vi "Autonomous Independent.vi"() -> ()   [LabVIEW 2016]
doc: "This VI is called when autonomous begins, and will automatically be terminated when autonomous ends. You can carry out timed or sensor driven robot movement independently without needing to return to the caller."
uses:
  Systems/Global 1.vi
  <vilib>/Rock Robotics/Network Tables/NT Read Number.vi
  Auto_Action.ctl
panel:
  in  "Oscillate effort":dbl=0.25 format="%#_13g"
  out "Auto Mode":dbl=10.0
  in  "Auton_Modes":T2(array[cluster])=[{"Actions"=[{"Effort"=0.55, "Duration"=3.5, "Action"=enum."Nothing", "Encoder"=0.0, "Condition"=FALSE}, {"Effort"=0.0, "Duration"=0.0, "Action"=enum."Nothing", "Encoder"=0.0, "Condition"=FALSE}]}, {"Actions"=[{"Effort"=0.53, "Duration"=1.0, "Action"=enum."Shoot", "Encoder"=6.462, "Condition"=TRUE}, {"Effort"=0.0, "Duration"=3.0, "Action"=enum."Index", "Encoder"=0.0, "Condition"=FALSE}, {"Effort"=0.3, "Duration"=2.0, "Action"=enum."Turn", "Encoder"=38.0, "Condition"=FALSE}, {"Effort"=0.3, "Duration"=5.0, "Action"=enum."Drive", "Encoder"=0.0, "Condition"=TRUE}, {"Effort"=0.25, "Duration"=0.0, "Action"=enum."Nothing", "Encoder"=57.0, "Condition"=FALSE}, {"Effort"=-0.25, "Duration"=0.0, "Action"=enum."Nothing", "Encoder"=0.0, "Condition"=FALSE}, {"Effort"=1.0, "Duration"=0.0, "Action"=enum."Nothing", "Encoder"=0.0, "Condition"=FALSE}, {"Effort"=0.25, "Duration"=0.0, "Action"=enum."Nothing", "Encoder"=0.0, "Condition"=FALSE}]}, {"Actions"=[{"Effort"=0.0, "Duration"=0.1, "Action"=enum."Drive Encoder Reset", "Encoder"=0.0, "Condition"=FALSE}, {"Effort"=0.0, "Duration"=1.0, "Action"=enum."Gyro Reset", "Encoder"=0.0, "Condition"=FALSE}, {"Effort"=0.3, "Duration"=2.5, "Action"=enum."Drive", "Encoder"=1000.0, "Condition"=TRUE}, {"Effort"=1.0, "Duration"=1.0, "Action"=enum."Gear0", "Encoder"=0.0, "Condition"=FALSE}, {"Effort"=1.0, "Duration"=0.0, "Action"=enum."Nothing", "Encoder"=0.0, "Condition"=FALSE}, {"Effort"=1.0, "Duration"=0.5, "Action"=enum."Nothing", "Encoder"=0.0, "Condition"=FALSE}, {"Effort"=0.0, "Duration"=0.0, "Action"=enum."Drive Encoder Reset", "Encoder"=0.0, "Condition"=FALSE}, {"Effort"=0.3, "Duration"=0.5, "Action"=enum."Nothing", "Encoder"=24.0, "Condition"=TRUE}, {"Effort"=0.0, "Duration"=0.0, "Action"=enum."Nothing", "Encoder"=0.0, "Condition"=FALSE}, {"Effort"=-0.2, "Duration"=2.0, "Action"=enum."Drive", "Encoder"=24.0, "Condition"=TRUE}, {"Effort"=0.0, "Duration"=0.0, "Action"=enum."Drive Encoder Reset", "Encoder"=0.0, "Condition"=FALSE}, {"Effort"=-0.25, "Duration"=0.0, "Action"=enum."Nothing", "Encoder"=12.0, "Condition"=FALSE}]}, {"Actions"=[{"Effort"=0.0, "Duration"=0.1, "Action"=enum."Drive Encoder Reset", "Encoder"=6.462, "Condition"=FALSE}, {"Effort"=0.0, "Duration"=0.1, "Action"=enum."Gyro Reset", "Encoder"=0.0, "Condition"=FALSE}, {"Effort"=-0.25, "Duration"=1.0, "Action"=enum."Drive", "Encoder"=6.462, "Condition"=FALSE}, {"Effort"=0.0, "Duration"=0.1, "Action"=enum."Gyro Reset", "Encoder"=0.0, "Condition"=FALSE}, {"Effort"=-0.25, "Duration"=0.0, "Action"=enum."Turn", "Encoder"=0.0, "Condition"=FALSE}, {"Effort"=-0.25, "Duration"=0.0, "Action"=enum."Drive", "Encoder"=7.5, "Condition"=FALSE}, {"Effort"=-1.0, "Duration"=0.0, "Action"=enum."Gear0", "Encoder"=0.0, "Condition"=FALSE}, {"Effort"=0.25, "Duration"=0.0, "Action"=enum."Drive", "Encoder"=3.0, "Condition"=FALSE}]}, {"Actions"=[{"Effort"=0.0, "Duration"=0.1, "Action"=enum."Drive Encoder Reset", "Encoder"=6.462, "Condition"=FALSE}, {"Effort"=0.0, "Duration"=0.1, "Action"=enum."Gyro Reset", "Encoder"=0.0, "Condition"=FALSE}, {"Effort"=-0.25, "Duration"=1.0, "Action"=enum."Drive", "Encoder"=6.462, "Condition"=FALSE}, {"Effort"=0.0, "Duration"=0.1, "Action"=enum."Gyro Reset", "Encoder"=0.0, "Condition"=FALSE}, {"Effort"=-0.25, "Duration"=0.0, "Action"=enum."Turn", "Encoder"=0.0, "Condition"=FALSE}, {"Effort"=-0.25, "Duration"=0.0, "Action"=enum."Drive", "Encoder"=7.5, "Condition"=FALSE}, {"Effort"=-1.0, "Duration"=0.0, "Action"=enum."Gear0", "Encoder"=0.0, "Condition"=FALSE}, {"Effort"=0.25, "Duration"=0.0, "Action"=enum."Drive", "Encoder"=3.0, "Condition"=FALSE}]}, {"Actions"=[{"Effort"=0.0, "Duration"=0.1, "Action"=enum."Drive Encoder Reset", "Encoder"=0.0, "Condition"=FALSE}, {"Effort"=0.0, "Duration"=0.1, "Action"=enum."Gyro Reset", "Encoder"=0.0, "Condition"=FALSE}, {"Effort"=0.25, "Duration"=1.0, "Action"=enum."Drive", "Encoder"=6.462, "Condition"=FALSE}, {"Effort"=1.0, "Duration"=0.1, "Action"=enum."Gyro Reset", "Encoder"=0.0, "Condition"=FALSE}, {"Effort"=0.25, "Duration"=0.0, "Action"=enum."Turn", "Encoder"=0.0, "Condition"=FALSE}, {"Effort"=0.25, "Duration"=0.0, "Action"=enum."Drive", "Encoder"=7.5, "Condition"=FALSE}, {"Effort"=1.0, "Duration"=0.0, "Action"=enum."Gear0", "Encoder"=0.0, "Condition"=FALSE}, {"Effort"=-0.25, "Duration"=0.0, "Action"=enum."Drive", "Encoder"=3.0, "Condition"=FALSE}]}, {"Actions"=[{"Effort"=0.0, "Duration"=0.1, "Action"=enum."Nothing", "Encoder"=0.0, "Condition"=FALSE}, {"Effort"=0.0, "Duration"=0.1, "Action"=enum."Gyro Reset", "Encoder"=0.0, "Condition"=FALSE}, {"Effort"=0.25, "Duration"=5.0, "Action"=enum."Drive", "Encoder"=60000.0, "Condition"=TRUE}, {"Effort"=0.75, "Duration"=1.0, "Action"=enum."Nothing", "Encoder"=0.0, "Condition"=FALSE}, {"Effort"=0.0, "Duration"=1.0, "Action"=enum."Nothing", "Encoder"=0.0, "Condition"=FALSE}, {"Effort"=0.0, "Duration"=0.0, "Action"=enum."Nothing", "Encoder"=0.0, "Condition"=FALSE}]}, {"Actions"=[{"Effort"=0.0, "Duration"=0.5, "Action"=enum."Drive Encoder Reset", "Encoder"=0.0, "Condition"=FALSE}, {"Effort"=0.55, "Duration"=4.25, "Action"=enum."Gyro Reset", "Encoder"=0.0, "Condition"=FALSE}, {"Effort"=-0.5, "Duration"=0.0, "Action"=enum."Drive", "Encoder"=46.0, "Condition"=FALSE}, {"Effort"=0.3, "Duration"=1.0, "Action"=enum."Nothing", "Encoder"=0.0, "Condition"=FALSE}, {"Effort"=0.3, "Duration"=2.0, "Action"=enum."Vision Correction", "Encoder"=76.6, "Condition"=FALSE}, {"Effort"=-0.25, "Duration"=1.0, "Action"=enum."Drive", "Encoder"=18.5, "Condition"=TRUE}, {"Effort"=1.0, "Duration"=0.0, "Action"=enum."Gear0", "Encoder"=0.0, "Condition"=FALSE}, {"Effort"=0.3, "Duration"=1.3, "Action"=enum."Drive", "Encoder"=30.0, "Condition"=TRUE}, {"Effort"=0.0, "Duration"=0.0, "Action"=enum."Nothing", "Encoder"=0.0, "Condition"=FALSE}, {"Effort"=0.03, "Duration"=0.0, "Action"=enum."Turn", "Encoder"=0.0, "Condition"=FALSE}, {"Effort"=0.0, "Duration"=0.0, "Action"=enum."Drive", "Encoder"=0.0, "Condition"=FALSE}]}, {"Actions"=[{"Effort"=0.0, "Duration"=0.0, "Action"=enum."Nothing", "Encoder"=0.0, "Condition"=FALSE}]}, {"Actions"=[{"Effort"=0.0, "Duration"=2.5, "Action"=enum."Shoot", "Encoder"=0.0, "Condition"=FALSE}, {"Effort"=0.0, "Duration"=5.0, "Action"=enum."Index", "Encoder"=0.0, "Condition"=FALSE}, {"Effort"=0.25, "Duration"=3.5, "Action"=enum."Nothing", "Encoder"=88.0, "Condition"=FALSE}, {"Effort"=1.0, "Duration"=1.0, "Action"=enum."Nothing", "Encoder"=0.0, "Condition"=FALSE}, {"Effort"=1.0, "Duration"=1.0, "Action"=enum."Nothing", "Encoder"=0.0, "Condition"=FALSE}, {"Effort"=1.0, "Duration"=0.5, "Action"=enum."Nothing", "Encoder"=0.0, "Condition"=FALSE}, {"Effort"=0.0, "Duration"=0.0, "Action"=enum."Nothing", "Encoder"=0.0, "Condition"=FALSE}, {"Effort"=-0.25, "Duration"=0.0, "Action"=enum."Nothing", "Encoder"=3.0, "Condition"=FALSE}, {"Effort"=0.0, "Duration"=0.0, "Action"=enum."Nothing", "Encoder"=0.0, "Condition"=FALSE}, {"Effort"=0.25, "Duration"=0.0, "Action"=enum."Nothing", "Encoder"=24.0, "Condition"=FALSE}, {"Effort"=0.0, "Duration"=0.0, "Action"=enum."Nothing", "Encoder"=0.0, "Condition"=FALSE}, {"Effort"=-0.25, "Duration"=0.0, "Action"=enum."Nothing", "Encoder"=12.0, "Condition"=FALSE}]}, {"Actions"=[{"Effort"=0.0, "Duration"=0.1, "Action"=enum."Drive Encoder Reset", "Encoder"=0.0, "Condition"=FALSE}, {"Effort"=0.0, "Duration"=1.0, "Action"=enum."Gyro Reset", "Encoder"=0.0, "Condition"=FALSE}, {"Effort"=0.3, "Duration"=1.4, "Action"=enum."Drive", "Encoder"=88.0, "Condition"=TRUE}, {"Effort"=0.3, "Duration"=4.0, "Action"=enum."Turn", "Encoder"=2.0, "Condition"=FALSE}, {"Effort"=1.0, "Duration"=1.0, "Action"=enum."Nothing", "Encoder"=0.0, "Condition"=FALSE}, {"Effort"=1.0, "Duration"=0.5, "Action"=enum."Nothing", "Encoder"=0.0, "Condition"=FALSE}, {"Effort"=0.0, "Duration"=0.0, "Action"=enum."Nothing", "Encoder"=0.0, "Condition"=FALSE}, {"Effort"=-0.25, "Duration"=0.0, "Action"=enum."Nothing", "Encoder"=3.0, "Condition"=FALSE}, {"Effort"=0.0, "Duration"=0.0, "Action"=enum."Nothing", "Encoder"=0.0, "Condition"=FALSE}, {"Effort"=0.25, "Duration"=0.0, "Action"=enum."Nothing", "Encoder"=24.0, "Condition"=FALSE}, {"Effort"=0.0, "Duration"=0.0, "Action"=enum."Nothing", "Encoder"=0.0, "Condition"=FALSE}, {"Effort"=-0.25, "Duration"=0.0, "Action"=enum."Nothing", "Encoder"=12.0, "Condition"=FALSE}]}, {"Actions"=[{"Effort"=0.0, "Duration"=1.0, "Action"=enum."Drive Encoder Reset", "Encoder"=0.0, "Condition"=FALSE}, {"Effort"=0.0, "Duration"=1.0, "Action"=enum."Shoot", "Encoder"=0.0, "Condition"=FALSE}, {"Effort"=0.25, "Duration"=5.0, "Action"=enum."Index", "Encoder"=88.0, "Condition"=FALSE}, {"Effort"=1.0, "Duration"=1.0, "Action"=enum."Nothing", "Encoder"=0.0, "Condition"=FALSE}, {"Effort"=1.0, "Duration"=1.0, "Action"=enum."Nothing", "Encoder"=0.0, "Condition"=FALSE}, {"Effort"=1.0, "Duration"=0.5, "Action"=enum."Nothing", "Encoder"=0.0, "Condition"=FALSE}, {"Effort"=0.0, "Duration"=0.0, "Action"=enum."Nothing", "Encoder"=0.0, "Condition"=FALSE}, {"Effort"=-0.25, "Duration"=0.0, "Action"=enum."Nothing", "Encoder"=3.0, "Condition"=FALSE}, {"Effort"=0.0, "Duration"=0.0, "Action"=enum."Nothing", "Encoder"=0.0, "Condition"=FALSE}, {"Effort"=0.25, "Duration"=0.0, "Action"=enum."Nothing", "Encoder"=24.0, "Condition"=FALSE}, {"Effort"=0.0, "Duration"=0.0, "Action"=enum."Nothing", "Encoder"=0.0, "Condition"=FALSE}, {"Effort"=-0.25, "Duration"=0.0, "Action"=enum."Nothing", "Encoder"=12.0, "Condition"=FALSE}]}, {"Actions"=[{"Effort"=0.0, "Duration"=0.1, "Action"=enum."Drive Encoder Reset", "Encoder"=0.0, "Condition"=FALSE}, {"Effort"=0.0, "Duration"=1.0, "Action"=enum."Gyro Reset", "Encoder"=0.0, "Condition"=FALSE}, {"Effort"=0.3, "Duration"=1.4, "Action"=enum."Drive", "Encoder"=88.0, "Condition"=TRUE}, {"Effort"=0.3, "Duration"=4.0, "Action"=enum."Turn", "Encoder"=0.0, "Condition"=FALSE}, {"Effort"=1.0, "Duration"=1.0, "Action"=enum."Nothing", "Encoder"=0.0, "Condition"=FALSE}, {"Effort"=1.0, "Duration"=0.5, "Action"=enum."Nothing", "Encoder"=0.0, "Condition"=FALSE}, {"Effort"=0.0, "Duration"=0.0, "Action"=enum."Nothing", "Encoder"=0.0, "Condition"=FALSE}, {"Effort"=0.3, "Duration"=0.5, "Action"=enum."Nothing", "Encoder"=24.0, "Condition"=TRUE}, {"Effort"=0.0, "Duration"=0.0, "Action"=enum."Nothing", "Encoder"=0.0, "Condition"=FALSE}, {"Effort"=-0.2, "Duration"=2.0, "Action"=enum."Nothing", "Encoder"=24.0, "Condition"=TRUE}, {"Effort"=0.0, "Duration"=0.0, "Action"=enum."Nothing", "Encoder"=0.0, "Condition"=FALSE}, {"Effort"=-0.25, "Duration"=0.0, "Action"=enum."Nothing", "Encoder"=12.0, "Condition"=FALSE}]}]
  # "Nothing"
  # "Boiler Right Right side gear"
  # "Middle Gear"
  # "Boiler Right Left Side Gear"
  # "Boiler Left RightSide Gear"
  # "Boiler Left Left Side Gear"
  # "Drive"
  # "Vision Correction"
  # "Hopper"
  # "10 ball"
  # "Farside"
  # "Boilerside-10 ball"
  # "Auto 5"
  # "Auto 6"
  # "Auto 6"
  # "Auto 7"
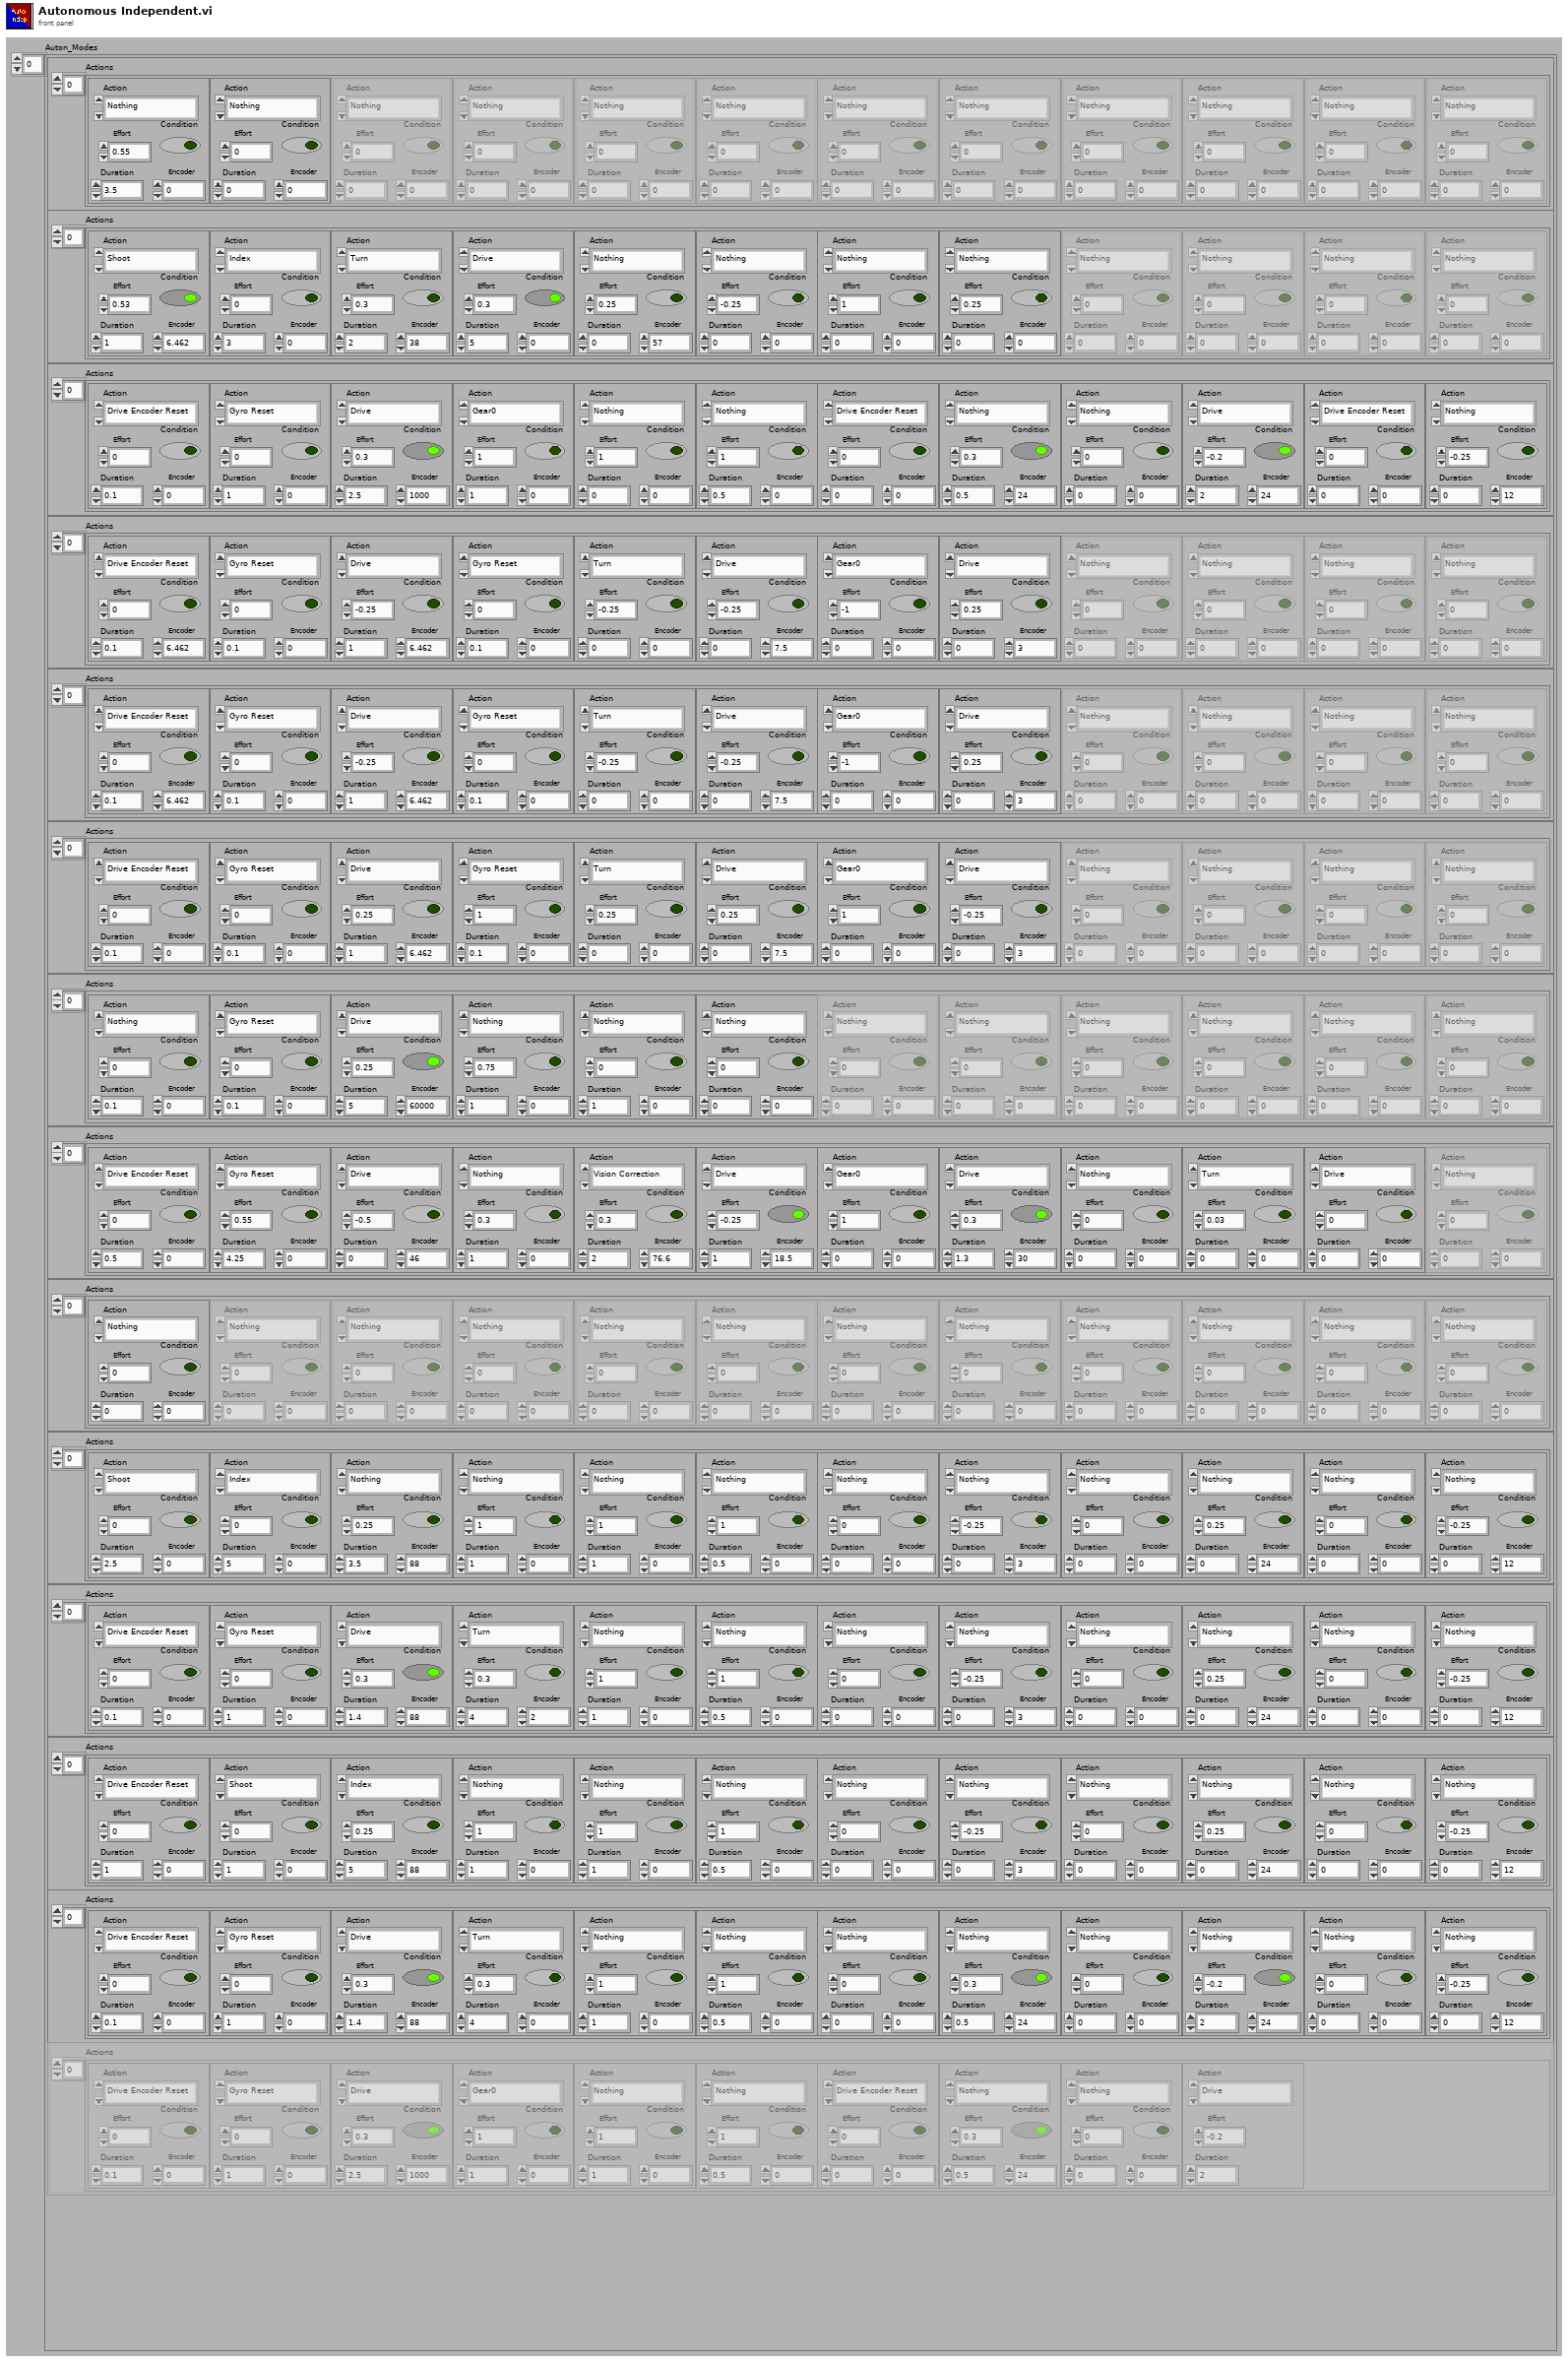
[diagram p1: front panel]
types:
  T1 = typedef "Auto_Action.ctl" = enum16{"Nothing", "Drive", "Vision Correction", "Turn", "Gear0", "Gear1", "Climb", "Intake", "Index", "Shoot", "Test", "Drive Encoder Reset", "Gyro Reset"}
  T2 = cluster{"Actions":cluster{"Effort":dbl, "Duration":dbl, "Action":T1, "Encoder":dbl, "Condition":bool}[]}[]
  T3 = cluster{"Actions":cluster{"Effort":dbl, "Duration":dbl, "Action":T1, "Encoder":dbl, "Condition":bool}[]}
  T4 = cluster{"Effort":dbl, "Duration":dbl, "Action":T1, "Encoder":dbl, "Condition":bool}[]
  T5 = typedef "WPI_MotorControlDeviceRef.ctl" = cluster{"DeviceStatus":errorcluster, "Type":T6, "PWM":cluster{"PWM Channel":T7, "DeadBand":T8}, "CAN":cluster{"Device Number":u8, "SetOutput VI Ref":variant, "GetOutput VI Ref":variant, "Enable VI Ref":variant, "Disable VI Ref":variant, "Data":variant}, "Invert":bool}
  T6 = typedef "WPI_MotorControlType.ctl" = enum16{"PWM", "CAN"}
  T7 = typedef "FPGA_DIOPWMChannel.ctl" = enum8{"PWM 0", "PWM 1", "PWM 2", "PWM 3", "PWM 4", "PWM 5", "PWM 6", "PWM 7", "PWM 8", "PWM 9", "PWM MXP 0", "PWM MXP 1", "PWM MXP 2", "PWM MXP 3", "PWM MXP 4", "PWM MXP 5", "PWM MXP 6", "PWM MXP 7", "PWM MXP 8", "PWM MXP 9", "Invalid"}
  T8 = typedef "WPI_PWMDeadband.ctl" = cluster{"Name":string, "maxPositivePwm":i32, "minPositivePwm":i32, "centerPwm":i32, "maxNegativePwm":i32, "minNegativePwm":i32, "angularRange":u16}
  T9 = typedef "WPI_CANTalonSRX_GlobalStatus.ctl" = cluster{"Applied Throttle":dbl, "Module Enabled":bool, "CAN Error":errorcluster, "Closed Loop Error":dbl, "Forward Limit Switch Closed":bool, "Reverse Limit Switch Closed":bool, "Sensor Position":dbl, "Sensor Velocity":dbl, "Current":dbl, "Sticky Fault - Over Temp":bool, "Sticky Fault - Under Voltage":bool, "Sticky Fault - Forward Limit":bool, "Sticky Fault - Reverse Limit":bool, "Sticky Fault - Forward Soft Limit":bool, "Sticky Fault - Reverse Soft Limit":bool, "Brake is Enabled":bool, "Encoder Position":dbl, "Encoder Velocity":dbl, "Encoder Index Count":dbl, "Encoder A Pin State":bool, "Encoder B Pin State":bool, "Encoder Index Pin State":bool, "Analog In":dbl, "Analog In Velocity":dbl, "Temperature (C)":dbl, "Battery Voltage":dbl, "Control 5 Is Supported":bool, "Current Profile Slot Select":dbl, "Pos Div 8":bool, "Vel Div 4":bool, "Pulse Width Position":i32, "Pulse Width Velocity":i32, "Pulse Width Rise To Rise (us)":i32, "Pulse Width Rise To Fall (us)":i32, "Mot Prof Active Is Under Run":bool, "Mot Prof Active Has Under Run":bool, "Mot Prof Active Is Last":bool, "Mot Prof Active Velocity Only":bool, "Mot Prof Active Is Valid":bool, "Mot Prof Buffer Is Full":bool, "Mot Prof Active Profile Slot Select":i32, "Mot Prof NextID":i32, "Mot Prof Count":i32, "Mot Prof Active Velocity":dbl, "Mot Prof Active Position":dbl, "Mot Prof Output Enable":i32}
  T10 = typedef "WPI_GyroDevRef.ctl" = cluster{"DevStatus":errorcluster, "Analog Channel":T11, "Offset":dbl, "Gain (VoltsPerDegree/Second)":dbl, "Gyro Type":enum16{"Analog", "XRS450"}, "Handle":i32, "SPI Bus":T12, "Device Found":bool, "Sample Rate":dbl, "Calibrate On Open":bool}
  T11 = typedef "FPGA_AIChannel.ctl" = enum8{"AI 0", "AI 1", "AI 2", "AI 3", "AI MXP 0", "AI MXP 1", "AI MXP 2", "AI MXP 3", "Invalid"}
  T12 = typedef "spi_bus.ctl" = enum16{"SPI On-Board, CS0", "SPI On-Board, CS1", "SPI On-Board, CS2", "SPI On-Board, CS3", "SPI MXP", "Invalid"}
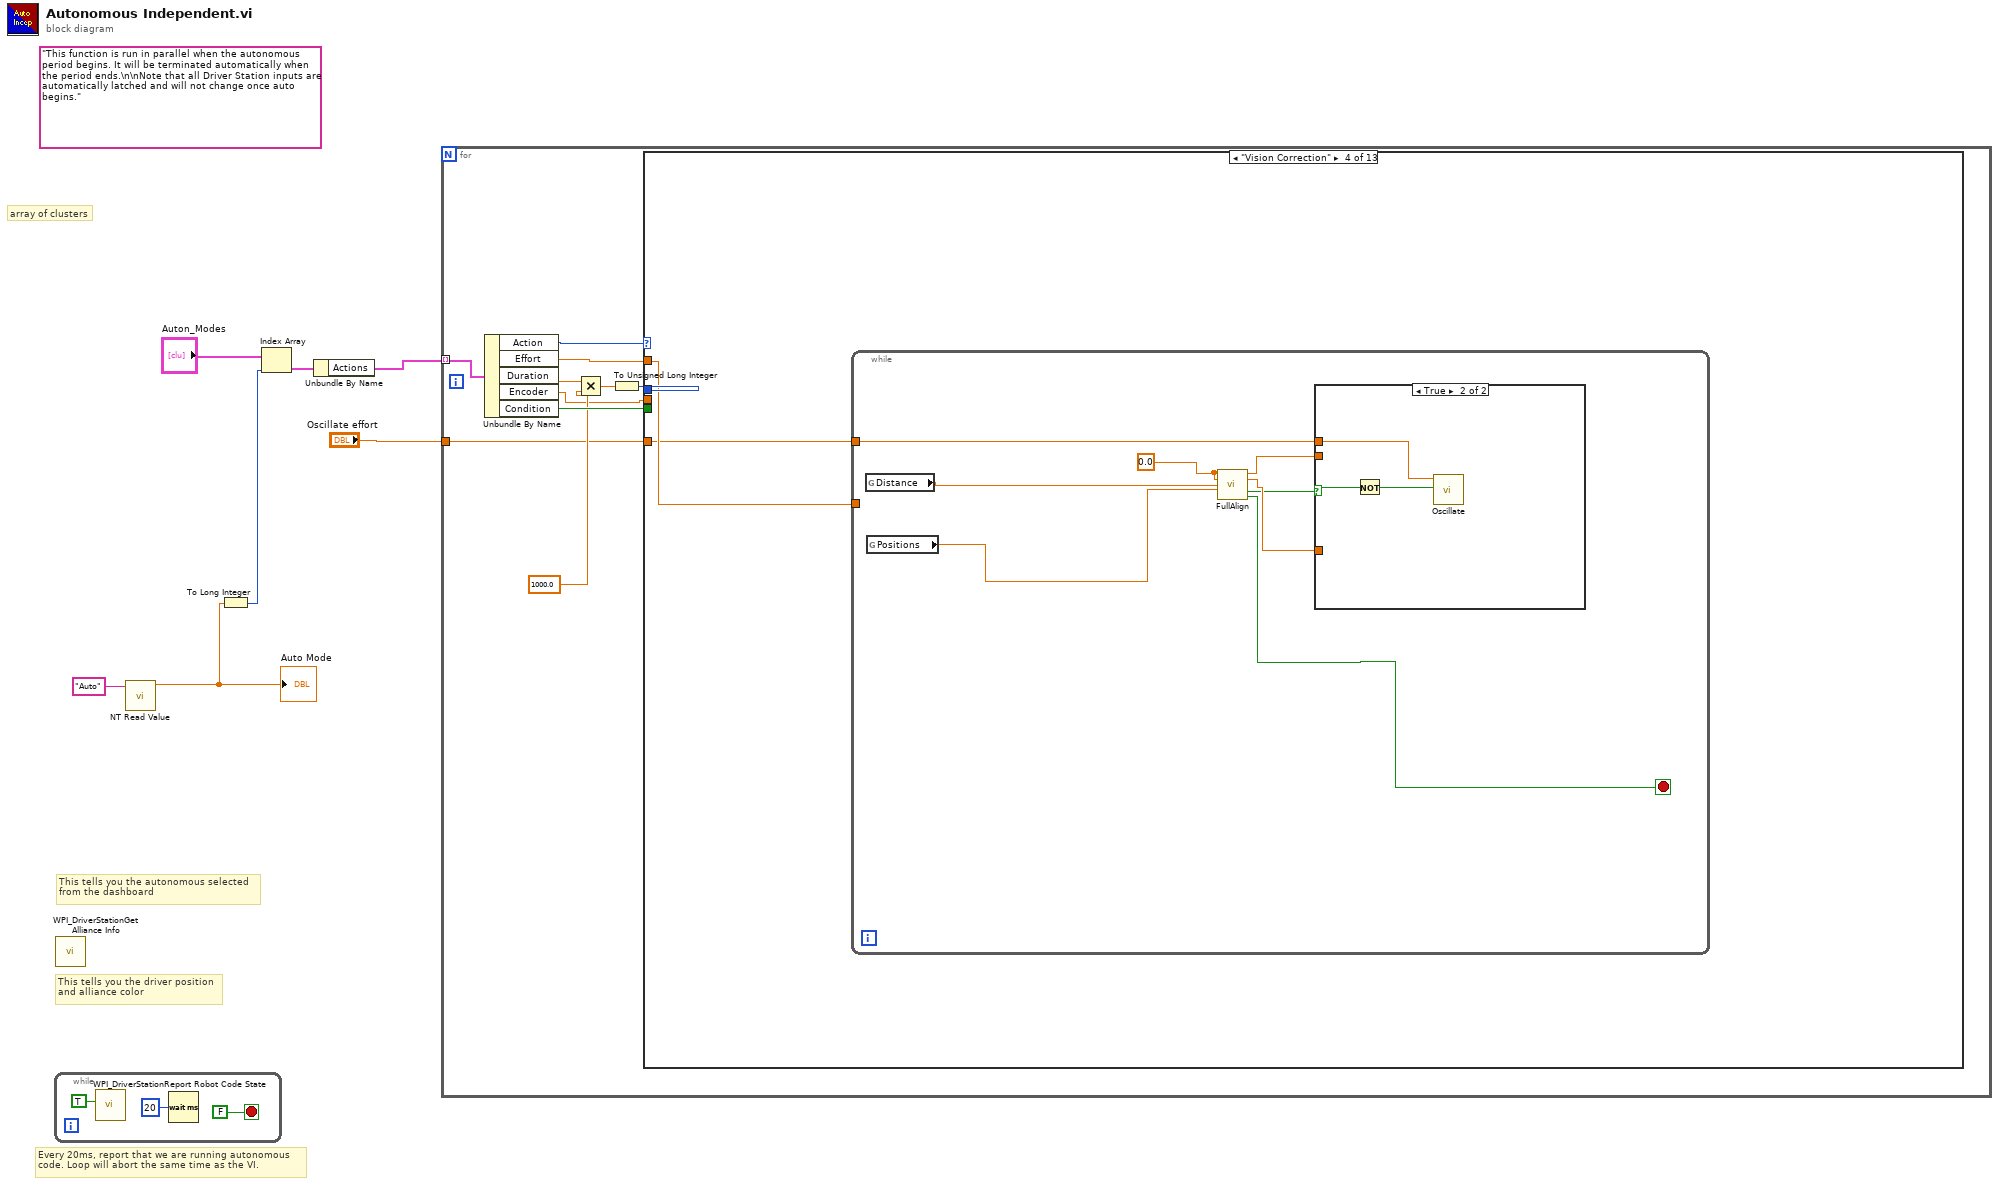
[diagram p0: block diagram]
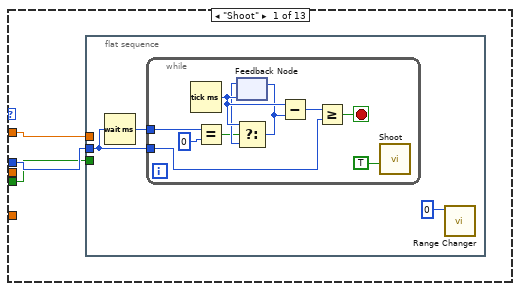
[diagram p2: hidden frame]
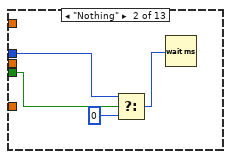
[diagram p3: hidden frame]
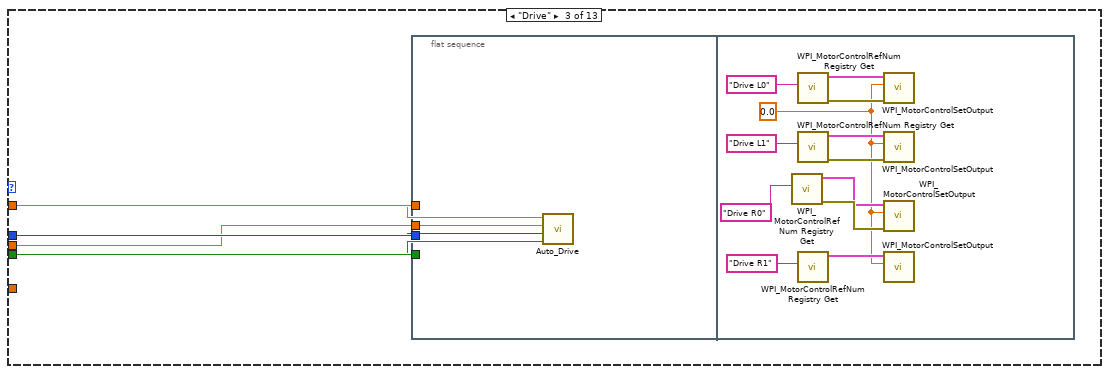
[diagram p4: hidden frame]
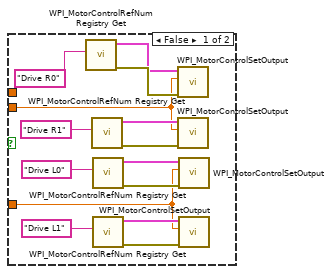
[diagram p5: hidden frame]
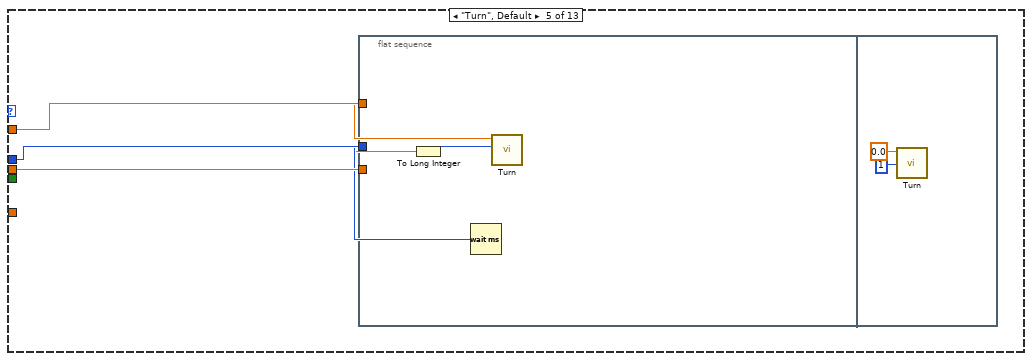
[diagram p6: hidden frame]
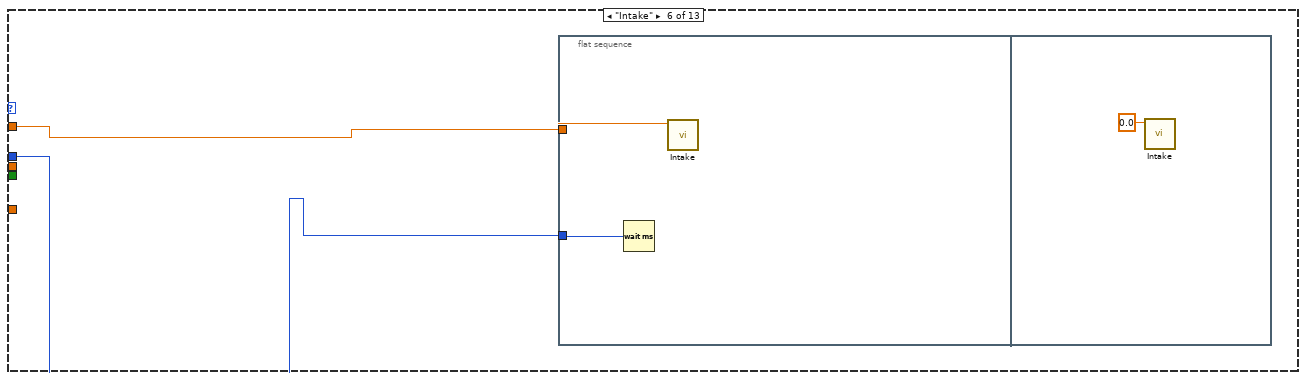
[diagram p7: hidden frame]
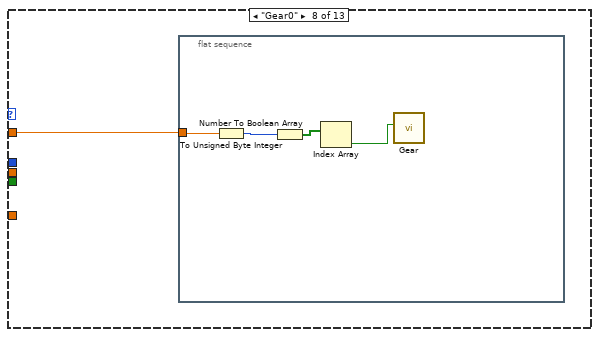
[diagram p9: hidden frame]
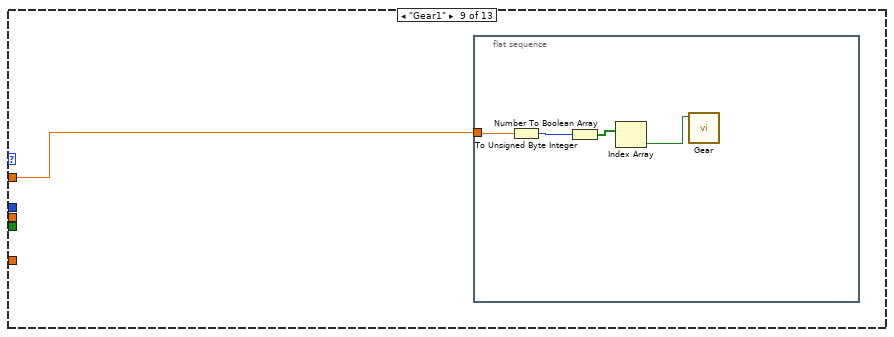
[diagram p10: hidden frame]
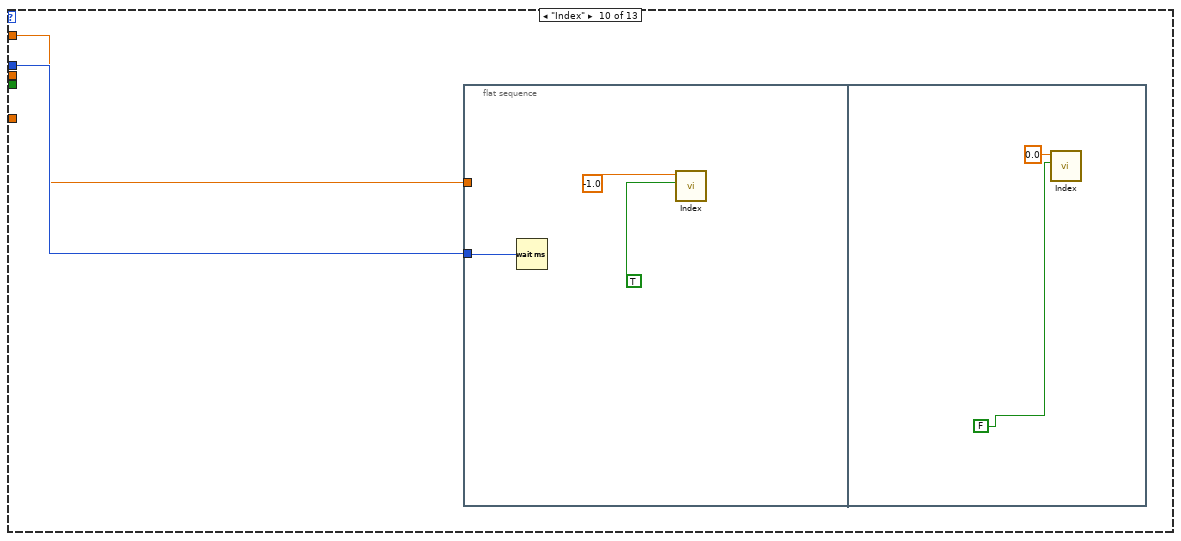
[diagram p11: hidden frame]
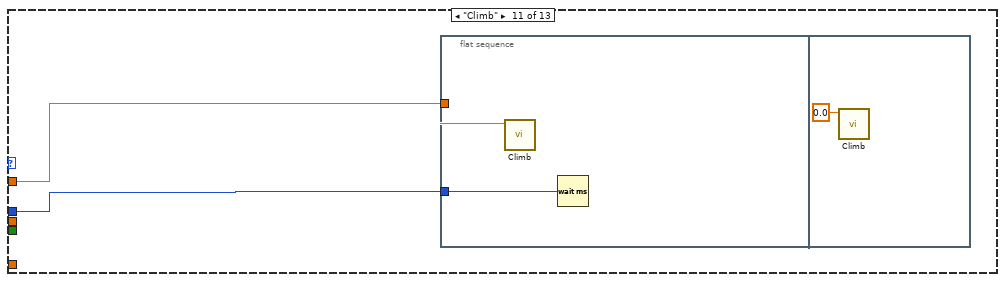
[diagram p12: hidden frame]
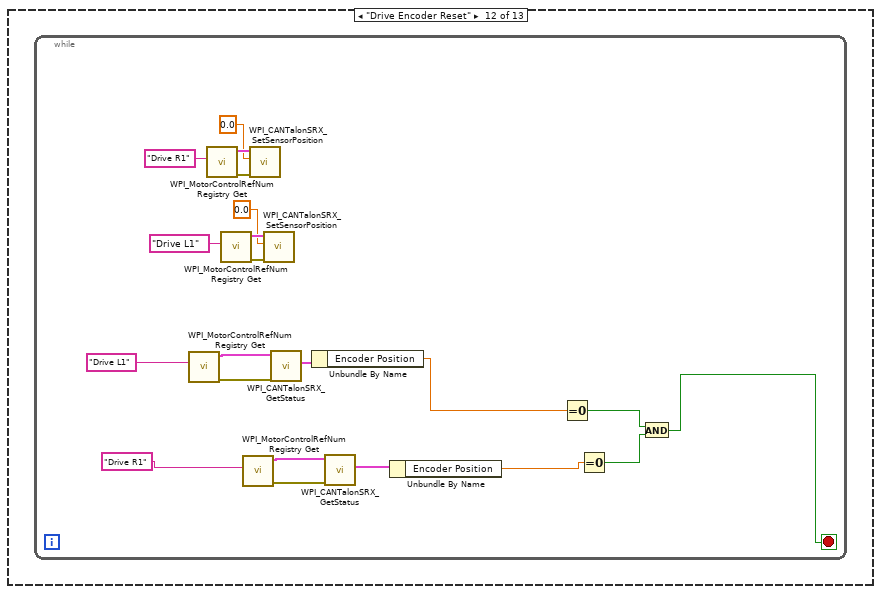
[diagram p13: hidden frame]
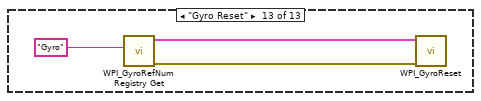
[diagram p14: hidden frame]
diagram:
  (unwired) "This function is run in parallel when the autonomous period begins. It will be terminated automatically when the period ends.\n\nNote that all Driver Station inputs are automatically latched and will not change once auto begins."
  # "This tells you the autonomous selected\nfrom the dashboard"
  # "array of clusters"
  # "Every 20ms, report that we are running autonomous\ncode. Loop will abort the same time as the VI."
  # "This tells you the driver position\nand alliance color"
  n1 = while {
    stop <- FALSE stop-if-true
    n2 = call <vilib>:"WPI_DriverStationReport Robot Code State.vi"("Autonomous"=TRUE) -> ()  [unwired: 10 in, 1 out]
    n3 = Wait (ms)(milliseconds to wait=u32 20) -> ()  [unwired: 1 out]
  }
  n4 = call <vilib>:"WPI_DriverStationGet Alliance Info.vi"() -> ()  [unwired: 12 out]
  n5 = call-poly <vilib>:"NT Read Value.vi"("Name"="Auto") -> ("Numeric"=w2:dbl)  [unwired: 9 in, 1 out]
  "Auto Mode" <- w2
  n6 = To Long Integer(number=w2) -> (32bit integer=w4:i32)
  n7 = Index Array(array="Auton_Modes", index=w4) -> (element=w6:T3)
  n8 = Unbundle By Name(w6) -> ("Actions"=w7:T4)
  n9 = for {
    tunnel: w7 -> [w20] mode=indexing
    tunnel: "Oscillate effort" -> [w11]
    n10 = Unbundle By Name(w20) -> ("Action"=w19:T1, "Effort"=w18:dbl, "Duration"=w17:dbl, "Encoder"=w12:dbl, "Condition"=w14:bool)
    n11 = Multiply(x=w17, y=1000.0) -> (x*y=w16:dbl)
    n12 = To Unsigned Long Integer(number=w16) -> (unsigned 32bit integer=w15:u32)
    n13 = case shown="\"Vision Correction\"" w19 {
      tunnel: w18 -> [w23 _ w44 w62 w90 w98 _ w102 w107 w112 w120 _ _]
      tunnel: w15 -> [w22 w39 w43 _ w89 w97 _ _ _ w113 w119 _ _]
      tunnel: w14 -> [w21 w40 w42 _ _ _ _ _ _ _ _ _ _]
      tunnel: w12 -> [_ _ w41 _ w88 _ _ _ _ _ _ _ _]
      tunnel: w11 -> [_ _ _ w61 _ _ _ _ _ _ _ _ _]
      frame "Shoot" {
        n14 = flat-sequence {
          tunnel: w23 -> [_]
          tunnel: w22 -> [w24]
          tunnel: w21 -> [_]
          frame #0 {
            n15 = Wait (ms)(milliseconds to wait=w24) -> (millisecond timer value=w25:u32)
            n16 = while {
              tunnel: w25 -> [w28]
              tunnel: w24 -> [w27]
              stop <- w29 stop-if-true
              n17 = Tick Count (ms)() -> (millisecond timer value=w35:u32)
              n18 = Equal?(x=w28, y=0) -> (x = y?=w33:bool)
              n19 = feedback #1(w35) -> (w34:u32)
              n20 = Select(t=w35, s=w33, f=w34) -> (s? t:f=w31:u32)
              n21 = feedback-in #1(w31) -> ()
              n22 = Subtract(x=w35, y=w31) -> (x-y=w30:u32)
              n23 = Greater Or Equal?(x=w30, y=w27) -> (x >= y?=w29:bool)
              n24 = call "Shoot.vi"("Shoot"=TRUE) -> ()  [unwired: 10 in]
            }
            n25 = call "Range Changer.vi"("POV"=i16 0) -> ()  [unwired: 10 in, 1 out]
          }
        }
      }
      frame "Nothing" {
        n26 = Select(t=w39, s=w40, f=u32 0) -> (s? t:f=w37:u32)
        n27 = Wait (ms)(milliseconds to wait=w37) -> ()  [unwired: 1 out]
      }
      frame "Drive" {
        n28 = flat-sequence {
          tunnel: w44 -> [w48]
          tunnel: w43 -> [w47]
          tunnel: w42 -> [w46]
          tunnel: w41 -> [w45]
          frame #0 {
            n29 = call "Auto_Drive.vi"("Timer?"=w46, "Duration"=w47, "distance"=w45, "Drive Effort"=w48) -> ()  [unwired: 8 in]
          }
          frame #1 {
            w49 = 0.0 ("Drive L")
            n30 = call <vilib>:"WPI_MotorControlRefNum Registry Get.vi"("refnum name"="Drive R0") -> ("error out"=w54:errorcluster, "MotorControlDevRef"=w50:T5)  [unwired: 9 in]
            n31 = call <vilib>:"WPI_MotorControlRefNum Registry Get.vi"("refnum name"="Drive L0") -> ("error out"=w55:errorcluster, "MotorControlDevRef"=w56:T5)  [unwired: 9 in]
            n32 = call <vilib>:"WPI_MotorControlRefNum Registry Get.vi"("refnum name"="Drive L1") -> ("error out"=w59:errorcluster, "MotorControlDevRef"=w58:T5)  [unwired: 9 in]
            n33 = call <vilib>:"WPI_MotorControlRefNum Registry Get.vi"("refnum name"="Drive R1") -> ("MotorControlDevRef"=w52:T5)  [unwired: 9 in, 1 out]
            n34 = call <vilib>:"WPI_MotorControlSetOutput.vi"("error in (no error)"=w55, "Output"=w49, "MotorControlDevRef"=w56) -> ()  [unwired: 6 in, 3 out]
            n35 = call <vilib>:"WPI_MotorControlSetOutput.vi"("error in (no error)"=w59, "Output"=w49, "MotorControlDevRef"=w58) -> ()  [unwired: 6 in, 3 out]
            n36 = call <vilib>:"WPI_MotorControlSetOutput.vi"("error in (no error)"=w54, "Output"=w49, "MotorControlDevRef"=w50) -> ()  [unwired: 6 in, 3 out]
            n37 = call <vilib>:"WPI_MotorControlSetOutput.vi"("Output"=w49, "MotorControlDevRef"=w52) -> ()  [unwired: 7 in, 3 out]
          }
        }
      }
      frame "Vision Correction" {
        n38 = while {
          tunnel: w62 -> [_]
          tunnel: w61 -> [w63]
          stop <- w65 stop-if-true
          w68 = 0.0
          n39 = global read "Global 1.vi" "Distance"() -> (w67:dbl)
          n40 = global read "Global 1.vi" "Positions"() -> (w66:dbl)
          n41 = call "FullAlign.vi"("Joystick 0"=w68, "Joystick 1"=w68, "Distance"=w67, "Angle"=w66) -> ("Right Motor"=w70:dbl, "Left Motor"=w69:dbl, "Not In Sight?"=w64:bool, "In Range?"=w65:bool)  [unwired: 8 in]
          n42 = case shown="True" w64 {
            selector: w64 -> [_ w87]
            tunnel: w70 -> [w72 _]
            tunnel: w69 -> [w71 _]
            tunnel: w63 -> [_ w85]
            frame False {
              n43 = call <vilib>:"WPI_MotorControlRefNum Registry Get.vi"("refnum name"="Drive R0") -> ("error out"=w78:errorcluster, "MotorControlDevRef"=w74:T5)  [unwired: 9 in]
              n44 = call <vilib>:"WPI_MotorControlRefNum Registry Get.vi"("refnum name"="Drive R1") -> ("error out"=w73:errorcluster, "MotorControlDevRef"=w76:T5)  [unwired: 9 in]
              n45 = call <vilib>:"WPI_MotorControlRefNum Registry Get.vi"("refnum name"="Drive L0") -> ("error out"=w79:errorcluster, "MotorControlDevRef"=w80:T5)  [unwired: 9 in]
              n46 = call <vilib>:"WPI_MotorControlRefNum Registry Get.vi"("refnum name"="Drive L1") -> ("error out"=w83:errorcluster, "MotorControlDevRef"=w82:T5)  [unwired: 9 in]
              n47 = call <vilib>:"WPI_MotorControlSetOutput.vi"("error in (no error)"=w78, "Output"=w72, "MotorControlDevRef"=w74) -> ()  [unwired: 6 in, 3 out]
              n48 = call <vilib>:"WPI_MotorControlSetOutput.vi"("error in (no error)"=w73, "Output"=w72, "MotorControlDevRef"=w76) -> ()  [unwired: 6 in, 3 out]
              n49 = call <vilib>:"WPI_MotorControlSetOutput.vi"("error in (no error)"=w79, "Output"=w71, "MotorControlDevRef"=w80) -> ()  [unwired: 6 in, 3 out]
              n50 = call <vilib>:"WPI_MotorControlSetOutput.vi"("error in (no error)"=w83, "Output"=w71, "MotorControlDevRef"=w82) -> ()  [unwired: 6 in, 3 out]
            }
            frame True {
              n51 = Not(x=w87) -> (.not. x?=w86:bool)
              n52 = call "Oscillate.vi"("Target In Sight?"=w86, "Effort"=w85) -> ()  [unwired: 10 in]
            }
          }
        }
      }
      frame "Turn", Default {
        n53 = flat-sequence {
          tunnel: w90 -> [w94]
          tunnel: w89 -> [w93]
          tunnel: w88 -> [w91]
          frame #0 {
            n54 = To Long Integer(number=w91) -> (32bit integer=w92:i32)
            n55 = Wait (ms)(milliseconds to wait=w93) -> ()  [unwired: 1 out]
            n56 = call "Turn.vi"("mode"=w92, "Effort"=w94) -> ()  [unwired: 10 in]
          }
          frame #1 {
            n57 = call "Turn.vi"("mode"=1, "Effort"=0.0) -> ()  [unwired: 10 in]
          }
        }
      }
      frame "Intake" {
        n58 = flat-sequence {
          tunnel: w98 -> [w100]
          tunnel: w97 -> [w99]
          frame #0 {
            n59 = Wait (ms)(milliseconds to wait=w99) -> ()  [unwired: 1 out]
            n60 = call "Intake.vi"("Effort"=w100) -> ()  [unwired: 11 in]
          }
          frame #1 {
            n61 = call "Intake.vi"("Effort"=0.0) -> ()  [unwired: 11 in]
          }
        }
      }
      frame "Test" {
      }
      frame "Gear0" {
        n62 = flat-sequence {
          tunnel: w102 -> [w106]
          frame #0 {
            n63 = To Unsigned Byte Integer(number=w106) -> (unsigned 8bit integer=w105:u8)
            n64 = Number To Boolean Array(number=w105) -> (Boolean array=w104:bool[])
            n65 = Index Array(array=w104) -> (element=w103:bool)  [unwired: 1 in]
            n66 = call "Gear.vi"("Gear0?"=w103) -> ()  [unwired: 11 in]
          }
        }
      }
      frame "Gear1" {
        n67 = flat-sequence {
          tunnel: w107 -> [w111]
          frame #0 {
            n68 = To Unsigned Byte Integer(number=w111) -> (unsigned 8bit integer=w110:u8)
            n69 = Number To Boolean Array(number=w110) -> (Boolean array=w109:bool[])
            n70 = Index Array(array=w109) -> (element=w108:bool)  [unwired: 1 in]
            n71 = call "Gear.vi"("Gear1?"=w108) -> ()  [unwired: 11 in]
          }
        }
      }
      frame "Index" {
        n72 = flat-sequence {
          tunnel: w113 -> [w114]
          tunnel: w112 -> [_]
          frame #0 {
            n73 = Wait (ms)(milliseconds to wait=w114) -> ()  [unwired: 1 out]
            n74 = call "Index.vi"("Shoot"=TRUE ("Override?"), "Output"=-1.0) -> ()  [unwired: 10 in]
          }
          frame #1 {
            n75 = call "Index.vi"("Shoot"=FALSE ("Override?"), "Output"=0.0) -> ()  [unwired: 10 in]
          }
        }
      }
      frame "Climb" {
        n76 = flat-sequence {
          tunnel: w120 -> [w122]
          tunnel: w119 -> [w121]
          frame #0 {
            n77 = call "Climb.vi"("Effort"=w122) -> ()  [unwired: 11 in]
            n78 = Wait (ms)(milliseconds to wait=w121) -> ()  [unwired: 1 out]
          }
          frame #1 {
            n79 = call "Climb.vi"("Effort"=0.0) -> ()  [unwired: 11 in]
          }
        }
      }
      frame "Drive Encoder Reset" {
        n80 = while {
          stop <- w124 stop-if-true
          n81 = call <vilib>:"WPI_MotorControlRefNum Registry Get.vi"("refnum name"="Drive L1") -> ("error out"=w134:errorcluster, "MotorControlDevRef"=w129:T5)  [unwired: 9 in]
          n82 = call <vilib>:"WPI_MotorControlRefNum Registry Get.vi"("refnum name"="Drive R1") -> ("error out"=w139:errorcluster, "MotorControlDevRef"=w138:T5)  [unwired: 9 in]
          n83 = call <vilib>:"WPI_MotorControlRefNum Registry Get.vi"("refnum name"="Drive L1") -> ("error out"=w141:errorcluster, "MotorControlDevRef"=w142:T5)  [unwired: 9 in]
          n84 = call <vilib>:"WPI_MotorControlRefNum Registry Get.vi"("refnum name"="Drive R1") -> ("error out"=w131:errorcluster, "MotorControlDevRef"=w130:T5)  [unwired: 9 in]
          n85 = call <vilib>:"WPI_CANTalonSRX_SetSensorPosition.vi"("error in (no error)"=w139, "New Sensor Position"=0.0, "CAN Talon SRX Ref"=w138) -> ()  [unwired: 7 in, 2 out]
          n86 = call <vilib>:"WPI_CANTalonSRX_SetSensorPosition.vi"("error in (no error)"=w141, "New Sensor Position"=0.0, "CAN Talon SRX Ref"=w142) -> ()  [unwired: 7 in, 2 out]
          n87 = call <vilib>:"WPI_CANTalonSRX_GetStatus.vi"("error in (no error)"=w134, "CAN Talon SRX Ref"=w129) -> ("Talon SRX Status"=w132:T9)  [unwired: 7 in, 2 out]
          n88 = Unbundle By Name(w132) -> ("Encoder Position"=w127:dbl)
          n89 = call <vilib>:"WPI_CANTalonSRX_GetStatus.vi"("error in (no error)"=w131, "CAN Talon SRX Ref"=w130) -> ("Talon SRX Status"=w133:T9)  [unwired: 7 in, 2 out]
          n90 = Unbundle By Name(w133) -> ("Encoder Position"=w128:dbl)
          n91 = Equal To 0?(x=w127) -> (x = 0?=w126:bool)
          n92 = Equal To 0?(x=w128) -> (x = 0?=w125:bool)
          n93 = And(x=w126, y=w125) -> (x .and. y?=w124:bool)
        }
      }
      frame "Gyro Reset" {
        n94 = call <vilib>:"WPI_GyroRefNum Registry Get.vi"("refnum name"="Gyro") -> ("error out"=w146:errorcluster, "GyroDevRef"=w147:T10)  [unwired: 9 in]
        n95 = call <vilib>:"WPI_GyroReset.vi"("error in"=w146, "GyroDevRef"=w147) -> ()  [unwired: 8 in, 2 out]
      }
    }
  }
